vi "LV to ITX  Retrieve Equation.vi"(0 "File or Folder Path":path, 1 "Data Type":T2, 5 "offset":i32, 7 "length":i32=1, 9 "index":T3={"a"=4, "b"=10, "c"=7, "d"=9, "f"=2, "N1"=2, "N2"=0, "N3"=0, "N4"=0, "g"=1}, 11 "formula (parameters: a,b,c,d,f,g). g = x":string="y1 = g;\ny2 = b;", 12 "Enum 2":T1, 13 "data index":i32, 14 "data length":i32=500) -> (4 "y1 vs g":cluster{dbl[], dbl[]}[](graph), 6 "y2 vs g":cluster{dbl[], dbl[]}[](graph), 8 "2D":dbl[][](graph), 10 "N":T4={"N1"=73.16571153186332, "N2"=3605738918.935894, "N3"=3605738918.935894, "N4"=3605738918.935894} {"N4" format="%#_6p"; "N3" format="%#_6p"; "N2" format="%#_6p"; "N1" format="%#_6p"}, 15 "Notes":string)   [LabVIEW 2019, in "LV-Data.ITX.lvclass"]
uses:
  LV-Data.ITX.lvclass
  <vilib>/Utility/miscctls.llb/LVOffsetAndMultiplierTypeDef.ctl
  Typedefs/Retrieve N Results.ctl
  Typedefs/Retrieve Index.ctl
  Typedefs/Retrieve Data Type.ctl
  Typedefs/Retrieve Formula Type.ctl
  <vilib>/gmath/NI_Gmath.lvlib
  LV-Data/LV-Data.lvclass
  <userlib>/LevyLab/Graph Utilities/graph_utilities.lvclass
panel:
  in  "error in":errorcluster
  in  "2D graph:\non = y1\noff = y2":bool=TRUE
  in  "D  is time?":bool
  in  "B is time?":bool
  out "time":string[][](table)
  in  "Use Folder Index File?":bool
  in  "Generate Folder Index File?":bool
  in  "Ez name":string="Ez name"
  in  "Ey name":string="Ey name"
  in  "Ex name":string="Ex name"
  in  "C y name":string="C y name"
  in  "D x name":string="D x name"
  in  "A y name":string="A y name"
  in  "B x name":string="B x name"
  out "Index, Wavenames":string[][](table)
  in  "recolor traces?":bool=TRUE
  in  "Ex":T5={"Offset"=0.0, "Multiplier"=1.0}
  in  "Ey":T5={"Offset"=0.0, "Multiplier"=1.0}
  out "Path":path
  out "counter":i32=9
  out "pattern":string="*.itx"
  # "YOU CAN CHOOSE THE FORMULA TYPE:"
  # "EQUATION"
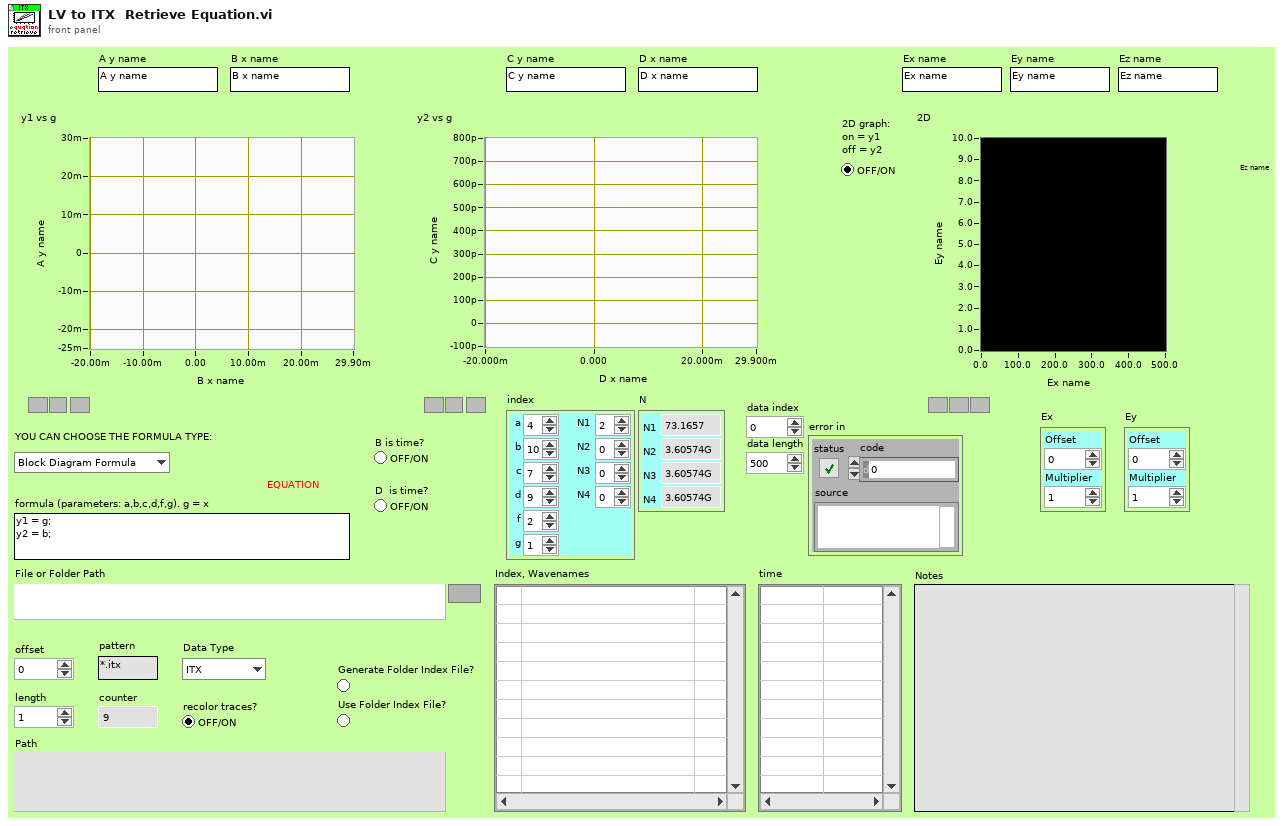
[diagram p1: front panel]
types:
  T1 = typedef "LV-Data.ITX.lvclass/Retrieve Formula Type.ctl" = enum16{"Block Diagram Formula", "String Formula"}
  T2 = typedef "LV-Data.ITX.lvclass/Retrieve Data Type.ctl" = enum16{"ITX", "ITX w/ 2D", "DAT", "TDMS"}
  T3 = typedef "LV-Data.ITX.lvclass/Retrieve Index.ctl" = cluster{"a":i32, "b":i32, "c":i32, "d":i32, "f":i32, "N1":i32, "N2":i32, "N3":i32, "N4":i32, "g":i32}
  T4 = typedef "LV-Data.ITX.lvclass/Retrieve N Results.ctl" = cluster{"N1":dbl, "N2":dbl, "N3":dbl, "N4":dbl}
  T5 = typedef "LVOffsetAndMultiplierTypeDef.ctl" = cluster{"Offset":dbl, "Multiplier":dbl}
  T6 = typedef "LV-Data.lvclass/Dictionary--cluster.ctl" = cluster{"key":string, "value":variant}
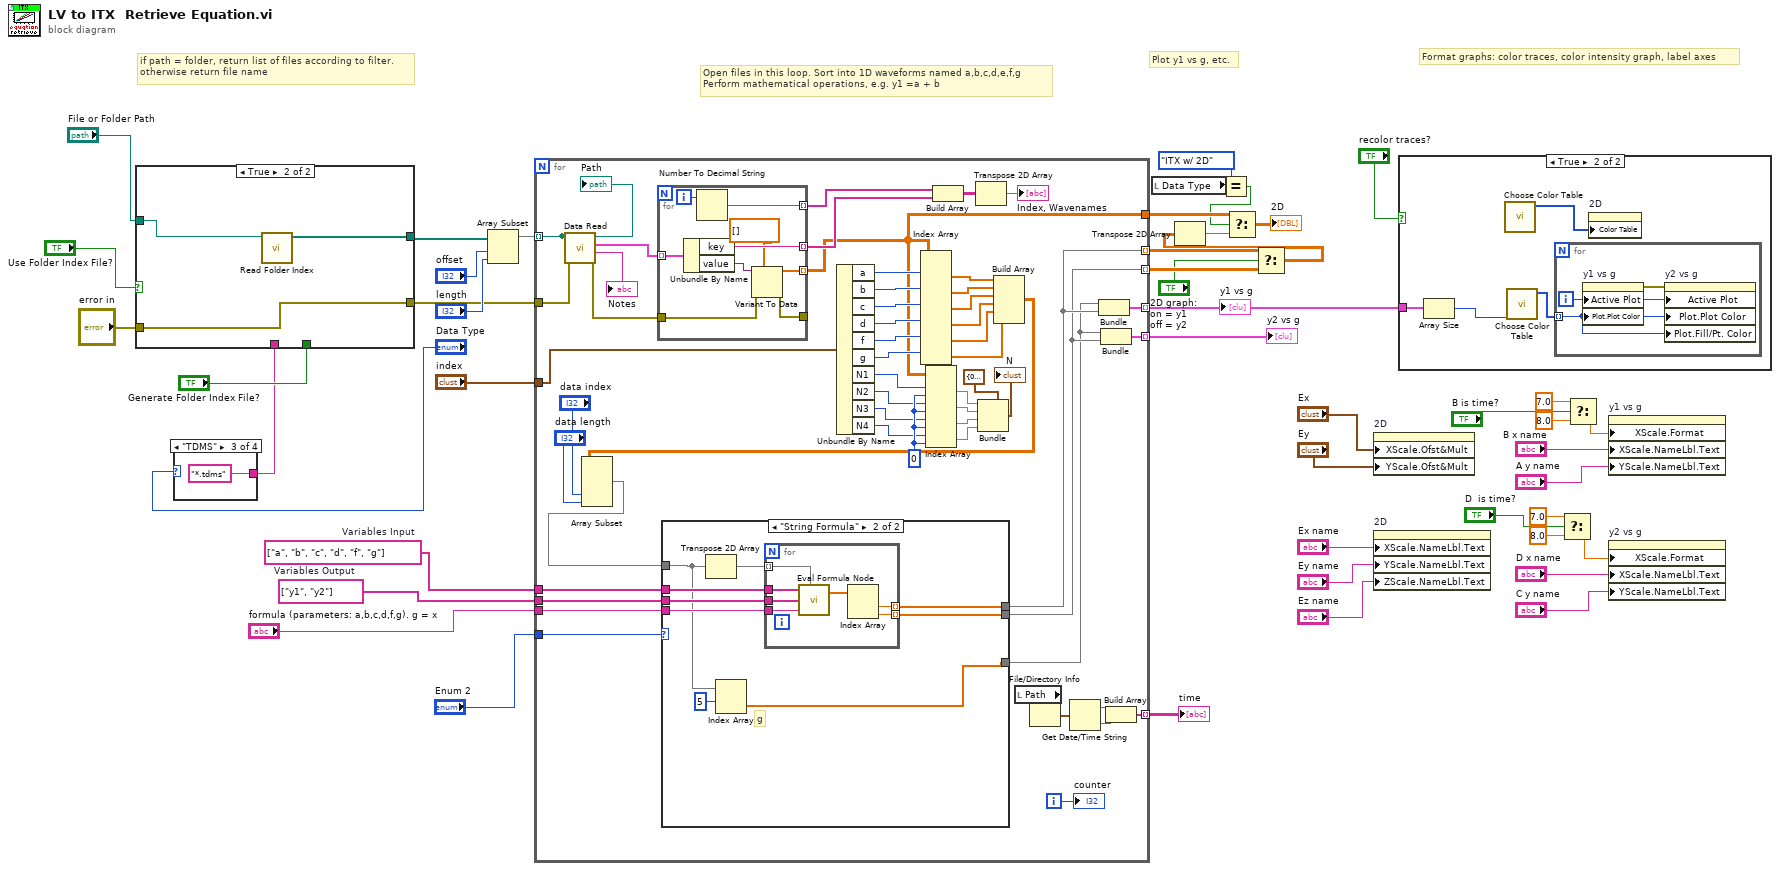
[diagram p0: block diagram]
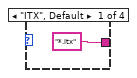
[diagram p2: hidden frame]
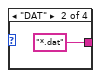
[diagram p3: hidden frame]
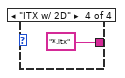
[diagram p4: hidden frame]
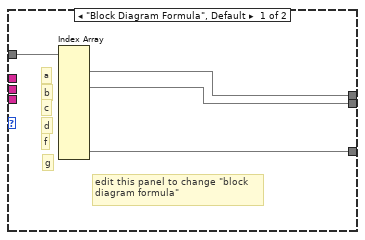
[diagram p6: hidden frame]
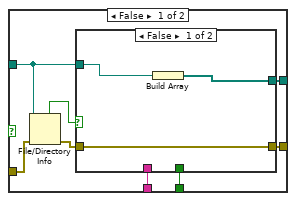
[diagram p7: hidden frame]
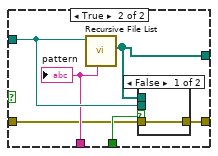
[diagram p8: hidden frame]
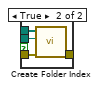
[diagram p9: hidden frame]
diagram:
  w13 = string[] ["a", "b", "c", "d", "f", "g"]  # Variables Input
  w6 = string[] ["y1", "y2"]  # Variables Output
  # "Plot y1 vs g, etc."
  # "Format graphs: color traces, color intensity graph, label axes"
  # "Open files in this loop. Sort into 1D waveforms named a,b,c,d,e,f,g\nPerform mathematical operations, e.g. y1 =a + b"
  # "if path = folder, return list of files according to filter.\notherwise return file name"
  n1 = case shown="\"TDMS\"" "Data Type" {
    tunnel: ["*.itx" ("pattern") "*.dat" ("pattern") "*.tdms" ("pattern") "*.itx" ("pattern")] -> w5
    frame "ITX", Default {
    }
    frame "DAT" {
    }
    frame "TDMS" {
    }
    frame "ITX w/ 2D" {
    }
  }
  n2 = case shown="True" "Use Folder Index File?" {
    tunnel: [w57 w75] -> w46
    tunnel: "File or Folder Path" -> [w59 w76]
    tunnel: "Generate Folder Index File?" -> [w56 _]
    tunnel: w5 -> [w55 _]
    tunnel: [w53 w74] -> w3
    tunnel: "error in" -> [w52 w74]
    frame False {
      n3 = File/Directory Info(path=w59, error in=w52) -> (directory=w58:bool, error out=w54:errorcluster)  [unwired: 5 out]
      n4 = case shown="False" w58 {
        tunnel: [w62 w64] -> w57
        tunnel: w59 -> [w61 w68]
        tunnel: w56 -> [_ w67]
        tunnel: w55 -> [_ w66]
        tunnel: w54 -> [w60 w65]
        tunnel: [w60 w63] -> w53
        frame False {
          n5 = Build Array(w61) -> (w62:path[])
        }
        frame True {
          n6 = call <vilib>:"Recursive File List.vi"("pattern"=w66, "Folder Path"=w68) -> ("All Files in Dir"=w64:path[])  [unwired: 5 in, 4 out]
          n7 = case shown="False" w67 {
            tunnel: w64 -> [_ w73]
            tunnel: w68 -> [_ w72]
            tunnel: w65 -> [w69 w71]
            tunnel: [w69 w70] -> w63
            frame False {
            }
            frame True {
              n8 = call "Create Folder Index.vi"("error in (no error)"=w71, "File or Folder Path"=w72, "All Files in Dir"=w73) -> ("error out"=w70:errorcluster)  [unwired: 8 in]
            }
          }
          "pattern" <- w66
        }
      }
    }
    frame True {
      n9 = call "Read Folder Index.vi"("File or Folder Path"=w76) -> ("Files"=w75:path[])  [unwired: 9 in, 1 out]
    }
  }
  n10 = Array Subset(array=w46, index="offset", length="length") -> (w27:path[])
  n11 = for {
    tunnel: w27 -> [w81] mode=indexing
    tunnel: [w81] -> _ mode=indexing
    tunnel: [w129] -> w15 mode=indexing
    tunnel: [w128] -> w38 mode=indexing
    tunnel: [w77] -> w40
    tunnel: [w116] -> w30 mode=indexing
    tunnel: "formula (parameters: a,b,c,d,f,g). g = x" -> [w110]
    tunnel: w6 -> [w109]
    tunnel: w13 -> [w108]
    tunnel: "index" -> [w89]
    tunnel: "Enum 2" -> [w107]
    tunnel: [w101] -> w11 mode=indexing
    tunnel: [w100] -> w9 mode=indexing
    tunnel: w3 -> [w80]
    i -> [w130]
    w125 = 0 ("disabled index (col)")
    n12 = call "Data Read.vi"("error in (no error)"=w80, "path"=w81) -> ("error out"=w82:errorcluster, "Notes"=→"Notes":string, "Data (Dictionary)"=w83:T6[], "path out"=→"Path":path)  [unwired: 6 in]
    n13 = for {
      tunnel: [w138] -> w79 mode=indexing
      tunnel: w83 -> [w137] mode=indexing
      tunnel: [w136] -> w78 mode=indexing
      tunnel: [w134] -> w77 mode=indexing
      tunnel: w82 -> [w132]
      tunnel: [w131] -> _
      i -> [w139]
      n14 = Unbundle By Name(w137) -> ("key"=w136:string, "value"=w133:variant)
      n15 = Number To Decimal String(number=w139) -> (decimal integer string=w138:string)  [unwired: 1 in]
      n16 = Variant To Data(error in=w132, type=dbl[] [], Variant=w133) -> (data=w134:dbl[], error out=w131:errorcluster)
    }
    n17 = Unbundle By Name(w89) -> ("a"=w124:i32, "b"=w123:i32, "c"=w122:i32, "d"=w121:i32, "f"=w111:i32, "g"=w88:i32, "N1"=w93:i32, "N2"=w92:i32, "N3"=w91:i32, "N4"=w90:i32)
    n18 = Index Array(array=w77, index (row) #1=w124, index (row) #2=w123, index (row) #3=w122, index (row) #4=w121, index (row) #5=w111, index (row) #6=w88) -> (element #1=w94:dbl[], element #2=w95:dbl[], element #3=w96:dbl[], element #4=w97:dbl[], element #5=w103:dbl[], element #6=w87:dbl[])  [unwired: 6 in]
    n19 = Index Array(array=w77, index (row) #1=w93, index (col) #1=w125, index (row) #2=w92, index (col) #2=w125, index (row) #3=w91, index (col) #3=w125, index (row) #4=w90, index (col) #4=w125) -> (element #1=w115:dbl, element #2=w114:dbl, element #3=w113:dbl, element #4=w112:dbl)
    n20 = Build Array(w79, w78) -> (w126:string[][])
    n21 = Transpose 2D Array(2D array=w126) -> (transposed array=→"Index, Wavenames":string[][])
    n22 = Bundle(cluster=cluster{"N1":dbl, "N2":dbl, "N3":dbl, "N4":dbl} {"N1"=0.0, "N2"=0.0, "N3"=0.0, "N4"=0.0}, "N1"=w115, "N2"=w114, "N3"=w113, "N4"=w112) -> (→"N":cluster{"N1":dbl, "N2":dbl, "N3":dbl, "N4":dbl})
    n23 = Build Array(w94, w95, w96, w97, w103, w87) -> (w99:dbl[][])
    n24 = Array Subset(array=w99, index (col)="data index", length (col)="data length") -> (w102:dbl[][])  [unwired: 2 in]
    n25 = case shown="\"String Formula\"" w107 {
      tunnel: [w142 w152] -> w100
      tunnel: w102 -> [w143 w146]
      tunnel: [w141 w151] -> w101
      tunnel: w110 -> [_ w150]
      tunnel: w109 -> [_ w149]
      tunnel: w108 -> [_ w148]
      tunnel: [w140 w144] -> w86
      frame "Block Diagram Formula", Default {
        # "g"
        # "f"
        # "d"
        # "c"
        # "b"
        # "a"
        # "edit this panel to change \"block\ndiagram formula\""
        n26 = Index Array(array=w143) -> (element #1=w141:dbl[], element #2=w142:dbl[], element #6=w140:dbl[])  [unwired: 12 in, 3 out]
      }
      frame "String Formula" {
        # "g"
        n27 = Transpose 2D Array(2D array=w146) -> (transposed array=w147:dbl[][])
        n28 = Index Array(array=w146, index (row)=5) -> (element=w144:dbl[])  [unwired: 1 in]
        n29 = for {
          tunnel: w148 -> [w159]
          tunnel: w149 -> [w158]
          tunnel: w150 -> [w157]
          tunnel: w147 -> [w153] mode=indexing
          tunnel: [w155] -> w152 mode=indexing
          tunnel: [w154] -> w151 mode=indexing
          n30 = call <vilib>:"Eval Formula Node.vi"("Variables Input"=w159, "Input Values"=w153, "Variables Output"=w158, "formula"=w157) -> ("Output Values"=w156:dbl[])  [unwired: 1 in, 1 out]
          n31 = Index Array(array=w156) -> (element #1=w154:dbl, element #2=w155:dbl)  [unwired: 2 in]
        }
      }
    }
    n32 = local read "Path"() -> (w120:path)
    n33 = File/Directory Info(path=w120) -> (last mod=w119:timestamp)  [unwired: 1 in, 6 out]
    n34 = Get Date/Time String(seconds (now)=w119) -> (date string=w118:string, time string=w117:string)  [unwired: 2 in]
    n35 = Bundle(w86, w101) -> (w129:cluster{dbl[], dbl[]})  [unwired: 1 in]
    n36 = Bundle(w86, w100) -> (w128:cluster{dbl[], dbl[]})  [unwired: 1 in]
    n37 = Build Array(w118, w117) -> (w116:string[])
    "counter" <- w130
  }
  "y1 vs g" <- w15
  "y2 vs g" <- w38
  "time" <- w30
  n38 = local read "Data Type"() -> (w17:T2)
  n39 = Equal?(x=enum16{"ITX", "ITX w/ 2D", "DAT"}."ITX w/ 2D" ("Enum"), y=w17) -> (x = y?=w16:bool)
  n40 = Select(t=w11, s="2D graph:\non = y1\noff = y2", f=w9) -> (s? t:f=w10:dbl[][])
  n41 = Transpose 2D Array(2D array=w10) -> (transposed array=w42:dbl[][])
  n42 = Select(t=w40, s=w16, f=w42) -> (s? t:f=→"2D":dbl[][])
  n43 = property on="2D" class="IntGraph (strict)"("XScale.Ofst&Mult"="Ex", "YScale.Ofst&Mult"="Ey") -> ()  [unwired: 2 in, 2 out]
  n44 = property on="2D" class="IntGraph (strict)"("XScale.NameLbl.Text"="Ex name", "YScale.NameLbl.Text"="Ey name", "ZScale.NameLbl.Text"="Ez name") -> ()  [unwired: 2 in, 2 out]
  n45 = case shown="True" "recolor traces?" {
    tunnel: w15 -> [_ w161]
    frame False {
    }
    frame True {
      n46 = Array Size(array=w161) -> (size(s)=w160:i32)
      n47 = call <userlib>:"Choose Color Table.vi"() -> ("Color Table"=w163:u32[])  [unwired: 8 in, 3 out]
      n48 = call <userlib>:"Choose Color Table.vi"("Size (256)"=w160) -> ("Color Table"=w162:u32[])  [unwired: 7 in, 3 out]
      n49 = for {
        tunnel: w162 -> [w164] mode=indexing
        i -> [w165]
        n50 = property on="y1 vs g" class="XYGraph (strict)"("Active Plot"=w165, "Plot.Plot Color"=w164) -> (error out=w166:errorcluster)  [unwired: 2 in, 1 out]
        n51 = property on="y2 vs g" class="XYGraph (strict)"(error in=w166, "Active Plot"=w165, "Plot.Plot Color"=w164, "Plot.Fill/Pt. Color"=w164) -> ()  [unwired: 1 in, 2 out]
      }
      n52 = property on="2D" class="IntGraph (strict)"("Color Table"=w163) -> ()  [unwired: 2 in, 2 out]
    }
  }
  n53 = Select(t=7.0, s="D  is time?", f=8.0) -> (s? t:f=w23:dbl)
  n54 = Select(t=7.0, s="B is time?", f=8.0) -> (s? t:f=w24:dbl)
  n55 = property on="y1 vs g" class="XYGraph (strict)"("XScale.Format"=w24, "XScale.NameLbl.Text"="B x name", "YScale.NameLbl.Text"="A y name") -> ()  [unwired: 2 in, 2 out]
  n56 = property on="y2 vs g" class="XYGraph (strict)"("XScale.Format"=w23, "XScale.NameLbl.Text"="D x name", "YScale.NameLbl.Text"="C y name") -> ()  [unwired: 2 in, 2 out]
